vi "AutoDoc.vi"() -> ()   [LabVIEW 2019, in "ArgosLib.lvlib"]
uses:
  ArgosLib.lvlib
panel:
  in  "stop":bool
  out "Active Step":string
  out "Progress Label":string
  out "Progress Bar":dbl(slide) caption="Slide" scale=0.0..1.0
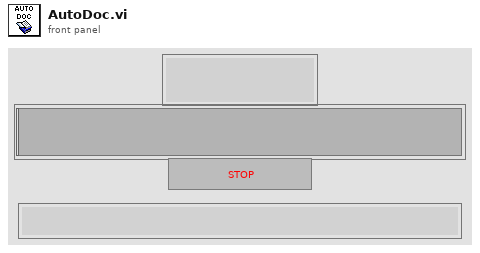
[diagram p1: front panel]
types:
  T1 = enum16{"open", "replace", "create", "open or create", "replace or create", "replace or create with confirmation"}
  T2 = enum32{"Custom", "Standard", "Using Panel", "Using SubVI", "Complete"}
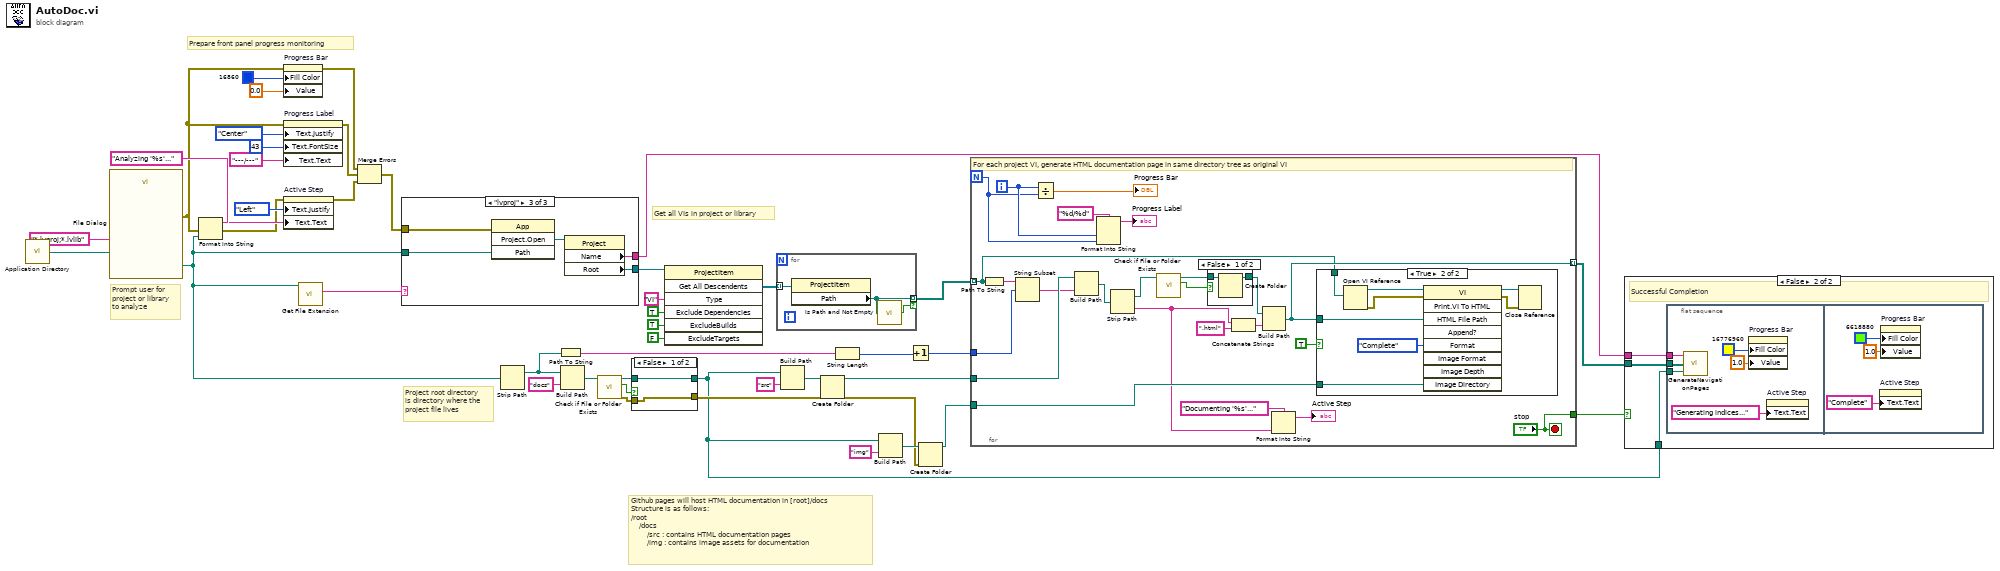
[diagram p0: block diagram]
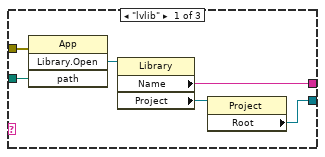
[diagram p2: hidden frame]
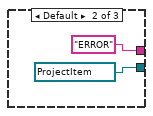
[diagram p3: hidden frame]
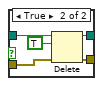
[diagram p4: hidden frame]
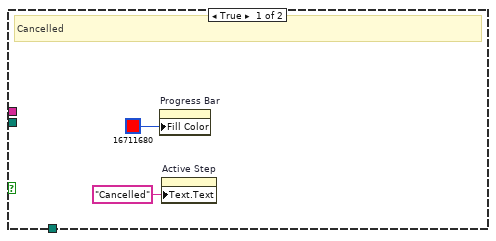
[diagram p5: hidden frame]
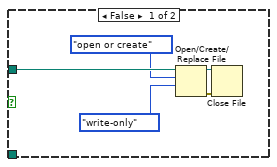
[diagram p6: hidden frame]
diagram:
  # "Prompt user for\nproject or library\nto analyze"
  # "Github pages will host HTML documentation in [root]/docs\nStructure is as follows:\n/root\n    /docs\n        /src : contains HTML documentation pages\n        /img : contains image assets for documentation"
  # "Project root directory\nis directory where the\nproject file lives"
  # "Get all VIs in project or library"
  # "Prepare front panel progress monitoring"
  n1 = call <vilib>:"Application Directory.vi"() -> ("Application Directory"=w41:path)
  n2 = call "File Dialog"("start path"=w41, "pattern (all files)"="*.lvproj;*.lvlib") -> ("selected path"=w2:path, "error out"=w17:errorcluster)  [unwired: 10 in, 2 out]
  n3 = Format Into String(format string="Analyzing '%s'...", error in=w17, w2) -> (resulting string=w22:string, error out=w19:errorcluster)  [unwired: 1 in]
  n4 = property on="Progress Bar" class="Slide (strict)"(error in=w17, "Fill Color"=u32 16860, "Value"=0.0 ("Progress Bar")) -> (error out=w14:errorcluster)  [unwired: 1 in, 1 out]
  n5 = property on="Progress Label" class="Str"(error in=w17, "Text.Justify"=enum16{"Left", "Center", "Right"}."Center" ("Text.Justification"), "Text.FontSize"=u32 43 ("Text.Font:Size"), "Text.Text"="---/---") -> (error out=w21:errorcluster)  [unwired: 1 in, 1 out]
  n6 = property on="Active Step" class="Str"(error in=w19, "Text.Justify"=enum16{"Left", "Center", "Right"}."Left" ("Text.Justification"), "Text.Text"=w22) -> (error out=w20:errorcluster)  [unwired: 1 in, 1 out]
  n7 = call <vilib>:"Get File Extension.vi"("file"=w2) -> ("lowercase file extension"=w1:string)  [unwired: 6 in, 4 out]
  n8 = Merge Errors(w14, w21, w20) -> (w18:errorcluster)
  n9 = case shown="\"lvproj\"" w1 {
    tunnel: [w49 refnum<vi> refnum ("Root") w58] -> w42
    tunnel: w18 -> [w52 _ w57]
    tunnel: [w47 "ERROR" ("Name") w56] -> w3
    tunnel: w2 -> [w51 _ w55]
    frame "lvlib" {
      n10 = invoke class="App" method="Library.Open"(error in=w52, "path"=w51) -> ("Open Library"=w50:refnum<vi>)  [unwired: 2 in, 3 out]
      n11 = property class="Library"(reference=w50) -> ("Name"=w47:string, "Project"=w48:refnum<vi>)  [unwired: 1 in, 2 out]
      n12 = property class="Project"(reference=w48) -> ("Root"=w49:refnum<vi>)  [unwired: 1 in, 2 out]
    }
    frame Default {
    }
    frame "lvproj" {
      n13 = invoke class="App" method="Project.Open"(error in=w57, "Path"=w55) -> ("Project:Open"=w59:refnum<vi>)  [unwired: 2 in, 3 out]
      n14 = property class="Project"(reference=w59) -> ("Name"=w56:string, "Root"=w58:refnum<vi>)  [unwired: 1 in, 2 out]
    }
  }
  n15 = Strip Path(path=w2) -> (stripped path=w31:path)  [unwired: 1 out]
  n16 = Path To String(path=w31) -> (string=w30:string)
  n17 = Build Path(base path=w31, name or relative path="docs") -> (appended path=w28:path)
  n18 = call <vilib>:"Check if File or Folder Exists.vi"("path"=w28) -> ("error out"=w8:errorcluster, "file or folder exists?"=w26:bool, "dup path"=w27:path)  [unwired: 8 in]
  n19 = case shown="False" w26 {
    tunnel: [w61 w65] -> w4
    tunnel: w27 -> [w61 w64]
    tunnel: w8 -> [w60 w63]
    tunnel: [w60 w62] -> w7
    frame False {
    }
    frame True {
      n20 = Delete(path (use dialog)=w64, entire hierarchy (F)=TRUE, error in=w63) -> (deleted path=w65:path, error out=w62:errorcluster)  [unwired: 2 in, 1 out]
    }
  }
  n21 = invoke class="ProjectItem" method="Get All Descendents"(reference=w42, "Type"="VI", "Exclude Dependencies"=TRUE ("ExcludeDependencies"), "ExcludeBuilds"=TRUE, "ExcludeTargets"=FALSE) -> ("All Descendents"=w39:refnum<vi>[])  [unwired: 2 in, 6 out]
  n22 = for {
    tunnel: w39 -> [w69] mode=indexing
    tunnel: [w68] -> w43 mode=indexing if=w67
    n23 = property class="ProjectItem"(reference=w69) -> ("Path"=w68:path)  [unwired: 1 in, 2 out]
    n24 = call <vilib>:"Is Path and Not Empty.vi"("path"=w68) -> ("Is Path and Not Empty?"=w67:bool)  [unwired: 4 in]
  }
  n25 = Build Path(base path=w4, name or relative path="src") -> (appended path=w11:path)
  n26 = Create Folder(path (use dialog)=w11, error in=w7) -> (created path=w10:path, error out=w6:errorcluster)  [unwired: 1 in, 1 out]
  n27 = String Length(string=w30) -> (length=w29:i32)
  n28 = Build Path(base path=w4, name or relative path="img") -> (appended path=w32:path)
  n29 = Increment(x=w29) -> (x+1=w45:i32)
  n30 = Create Folder(path (use dialog)=w32, error in=w6) -> (created path=w46:path)  [unwired: 1 in, 2 out]
  n31 = for {
    N -> [w78]
    tunnel: w46 -> [w91]
    tunnel: w43 -> [w70] mode=indexing
    tunnel: w10 -> [w88]
    tunnel: w45 -> [w89]
    tunnel: ["stop"] -> w44
    tunnel: [w72] -> w5 mode=indexing
    i -> [w79]
    stop <- "stop" stop-if-true
    # "For each project VI, generate HTML documentation page in same directory tree as original VI"
    n32 = Path To String(path=w70) -> (string=w90:string)
    n33 = String Subset(string=w90, offset (0)=w89) -> (substring=w87:string)  [unwired: 1 in]
    n34 = Divide(x=w79, y=w78) -> (x/y=→"Progress Bar":dbl)
    n35 = Build Path(base path=w88, name or relative path=w87) -> (appended path=w86:path)
    n36 = Format Into String(format string="%d/%d", w79, w78) -> (resulting string=→"Progress Label":string)  [unwired: 2 in, 1 out]
    n37 = Strip Path(path=w86) -> (stripped path=w84:path, name=w76:string)
    n38 = call <vilib>:"Check if File or Folder Exists.vi"("path"=w84) -> ("file or folder exists?"=w82:bool, "dup path"=w83:path)  [unwired: 8 in, 1 out]
    n39 = case shown="False" w82 {
      tunnel: [w108 w109] -> w85
      tunnel: w83 -> [w107 w109]
      frame False {
        n40 = Create Folder(path (use dialog)=w107) -> (created path=w108:path)  [unwired: 2 in, 2 out]
      }
      frame True {
      }
    }
    n41 = Concatenate Strings(w76, ".html" ("string")) -> (w92:string)
    n42 = Build Path(base path=w85, name or relative path=w92) -> (appended path=w72:path)
    n43 = Format Into String(format string="Documenting '%s'...", w76) -> (resulting string=→"Active Step":string)  [unwired: 2 in, 1 out]
    n44 = case shown="True" TRUE {
      tunnel: w91 -> [_ w105]
      tunnel: w72 -> [w98 w104]
      tunnel: w70 -> [_ w103]
      frame False {
        n45 = Open/Create/Replace File(file path (use dialog)=w98, operation (0:open)=T1."open or create", access (0:read/write)=enum16{"read/write", "read-only", "write-only"}."write-only") -> (refnum out=w97:refnum<file>, error out=w96:errorcluster)  [unwired: 3 in, 1 out]
        n46 = Close File(refnum=w97, error in=w96) -> ()  [unwired: 2 out]
      }
      frame True {
        n47 = Open VI Reference(vi path=w103) -> (vi reference=w101:refnum<vi>, error out=w102:errorcluster)  [unwired: 5 in]
        n48 = invoke class="VI" method="Print.VI To HTML"(reference=w101, error in=w102, "HTML File Path"=w104, "Format"=T2."Complete", "Image Directory"=w105) -> (reference out=w99:refnum<vi>, error out=w100:errorcluster)  [unwired: 4 in, 7 out]
        n49 = Close Reference(reference=w99, error in (no error)=w100) -> ()  [unwired: 1 out]
      }
    }
  }
  n50 = case shown="False" w44 {
    tunnel: w5 -> [_ w114]
    tunnel: w4 -> [_ w113]
    tunnel: w3 -> [_ w112]
    frame True {
      # "Cancelled"
      n51 = property on="Progress Bar" class="Slide (strict)"("Fill Color"=u32 16711680) -> ()  [unwired: 2 in, 2 out]
      n52 = property on="Active Step" class="Str"("Text.Text"="Cancelled") -> ()  [unwired: 2 in, 2 out]
    }
    frame False {
      # "Successful Completion"
      n53 = flat-sequence {
        tunnel: w114 -> [w117]
        tunnel: w113 -> [w116]
        tunnel: w112 -> [w115]
        frame #0 {
          n54 = call "GenerateNavigationPages.vi"("Root Directory"=w116, "VI Documentation Pages"=w117, "Project name"=w115) -> ()  [unwired: 2 in]
          n55 = property on="Progress Bar" class="Slide (strict)"("Fill Color"=u32 16776960, "Value"=1.0 ("Progress Bar")) -> ()  [unwired: 2 in, 2 out]
          n56 = property on="Active Step" class="Str"("Text.Text"="Generating indices...") -> ()  [unwired: 2 in, 2 out]
        }
        frame #1 {
          n57 = property on="Active Step" class="Str"("Text.Text"="Complete") -> ()  [unwired: 2 in, 2 out]
          n58 = property on="Progress Bar" class="Slide (strict)"("Fill Color"=u32 6618880, "Value"=1.0 ("Progress Bar")) -> ()  [unwired: 2 in, 2 out]
        }
      }
    }
  }
